vi "PXI-Pause-Wait for Underflow.vi"(0 "AO Tasks":T1[](array[typedef]), 7 "Abort?":bool, 9 "Pause?":bool, 11 "error in (no error)":errorcluster) -> (8 "Abort out":bool, 10 "Pause out":bool, 15 "error out":errorcluster)   [LabVIEW 2020]
uses:
  Type Defs/Task Struct.ctl
  PXI Globals.vi
  <resource>/objmgr/daqmx.rc
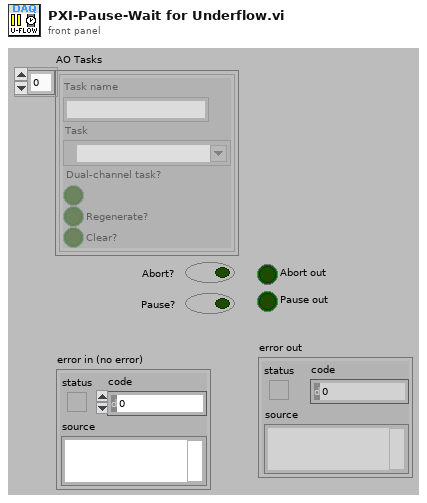
[diagram p1: front panel]
types:
  T1 = typedef "Task Struct.ctl" = cluster{"Task name":string, "Task":refnum<k21>, "Dual-channel task?":bool, "Regenerate?":bool, "Clear?":bool}
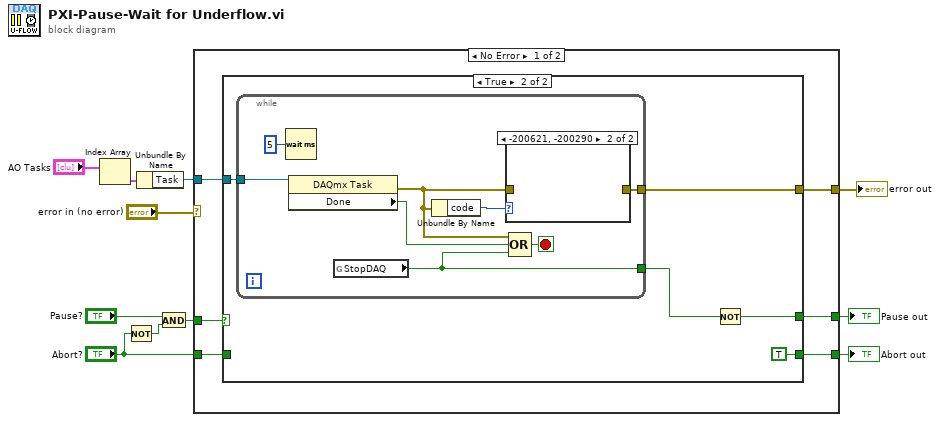
[diagram p0: block diagram]
diagram:
  n1 = Index Array(array="AO Tasks") -> (element=w9:T1)  [unwired: 1 in]
  n2 = Not(x="Abort?") -> (.not. x?=w5:bool)
  n3 = Unbundle By Name(w9) -> ("Task"=w7:refnum<k21>)
  n4 = And(x="Pause?", y=w5) -> (x .and. y?=w4:bool)
  n5 = case shown="No Error" "error in (no error)" {
    selector: "error in (no error)" -> [_ w34]
    tunnel: [w16 w34] -> w10
    tunnel: w7 -> [w17 _]
    tunnel: w4 -> [w15 _]
    tunnel: "Abort?" -> [w14 w33]
    tunnel: [w13 w33] -> w2
    tunnel: [w12 _] -> w1
    frame No Error {
      n6 = case shown="True" w15 {
        tunnel: w17 -> [_ w23]
        tunnel: [_ w22] -> w16
        tunnel: w14 -> [w18 _]
        tunnel: [w18 TRUE ("Abort?")] -> w13
        tunnel: [_ w20] -> w12
        frame False {
        }
        frame True {
          n7 = while {
            tunnel: w23 -> [w30]
            tunnel: [w26] -> w22
            tunnel: [w25] -> w21
            stop <- w29 stop-if-true
            n8 = Wait (ms)(milliseconds to wait=u32 5) -> ()  [unwired: 1 out]
            n9 = property class="DAQmx Task"(reference=w30) -> (error out=w24:errorcluster, "Done"=w28:bool)  [unwired: 1 in, 1 out]
            n10 = global read "PXI Globals.vi" "StopDAQ"() -> (w25:bool)
            n11 = Unbundle By Name(w24) -> ("code"=w27:i32)
            n12 = case shown="-200621, -200290" w27 {
              tunnel: w24 -> [w32 _]
              tunnel: [w32 _] -> w26
              frame 0, Default {
              }
              frame -200621, -200290 {
              }
            }
            n13 = Compound Arithmetic op=OR(w24, w28, w25) -> (w29:bool)
          }
          n14 = Not(x=w21) -> (.not. x?=w20:bool)
        }
      }
    }
    frame Error {
    }
  }
  "error out" <- w10
  "Abort out" <- w2
  "Pause out" <- w1
